vi "New.vi"(8 "Error In":errorcluster, 11 "Key":string) -> (0 "Error Out":errorcluster, 3 "Partial":refnum<class "Partial.lvclass">)   [LabVIEW 2017, in "Mustache.lvlib" / "Tokens.lvlib" / "Partial.lvclass"]
uses:
  Partial.lvclass
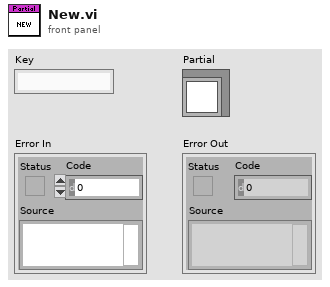
[diagram p1: front panel]
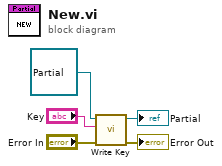
[diagram p0: block diagram]
diagram:
  n1 = call-dynamic "Write Key.vi"("Error In"="Error In", "Key"="Key", "Variable In"=refnum<class "Partial.lvclass"> refnum ("Mustache.lvlib:Tokens.lvlib:Partial.lvclass")) -> ("Error Out"=→"Error Out":errorcluster, "Variable Out"=→"Partial":refnum<class "Partial.lvclass">)  [unwired: 7 in]
